vi "Set Sender.vi"(10 "Sender":refnum<class "Sender.lvclass">, 11 "Setup Msg in":refnum<class "Setup Msg.lvclass">) -> (3 "Setup Msg out":refnum<class "Setup Msg.lvclass">)   [LabVIEW 2021, in "jettl.lvlib" / "Setup Msg.lvlib" / "Setup Msg.lvclass"]
uses:
  Setup Msg.lvclass
  Sender/Sender/Sender.lvclass
  Setup Msg.lvclass/Setup Msg.ctl
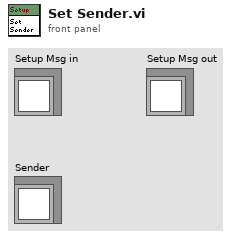
[diagram p1: front panel]
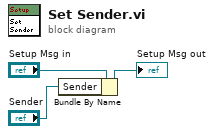
[diagram p0: block diagram]
diagram:
  n1 = Bundle By Name(cluster="Setup Msg in", "Sender"="Sender") -> (→"Setup Msg out":refnum<class "Setup Msg.lvclass">)
